vi "Find Region Indices.vi"(11 "Spreadsheet Array":string[][](array[string])) -> (0 "UES Index":i32[](array[numeric]), 1 "Hypo Index":i32[](array[numeric]), 2 "Tongue Index":i32[](array[numeric]), 3 "Velo Index":i32[](array[numeric]))   [LabVIEW 2020]
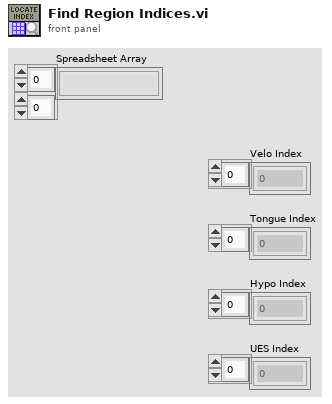
[diagram p1: front panel]
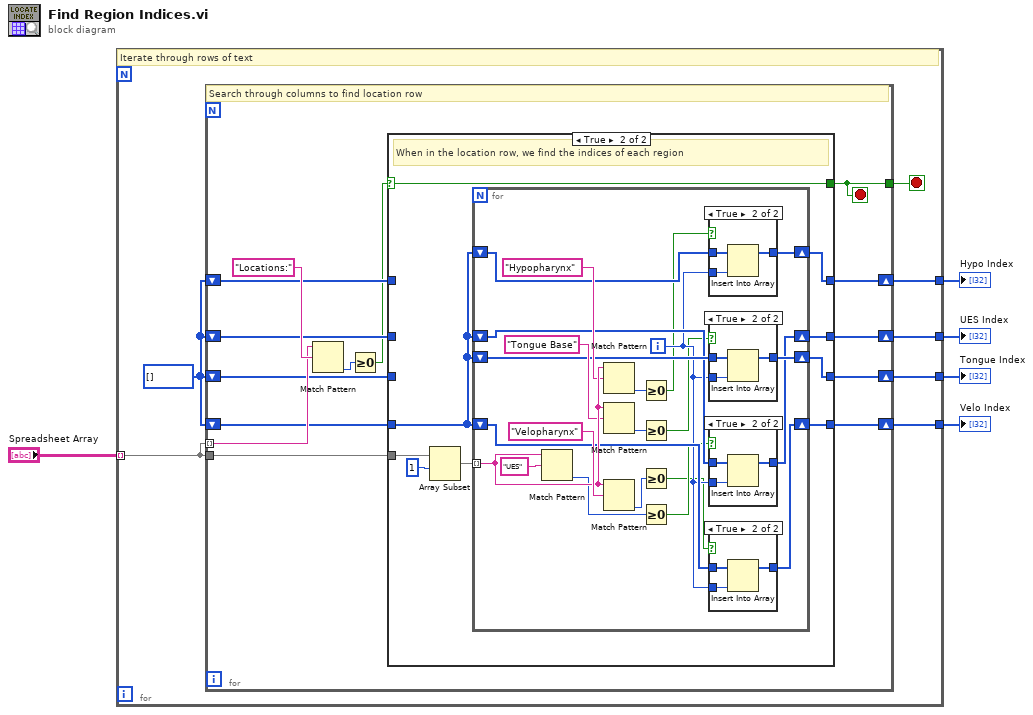
[diagram p0: block diagram]
diagram:
  n1 = for {
    tunnel: [w12] -> w5
    tunnel: [w11] -> w4
    tunnel: [w10] -> w3
    tunnel: [w9] -> w2
    tunnel: "Spreadsheet Array" -> [w7] mode=indexing
    stop <- w6 stop-if-true
    w8 = i32[] [] ("array")
    # "Iterate through rows of text"
    n2 = for {
      tunnel: w7 -> [w24] mode=indexing
      tunnel: w7 -> [w14]
      shift-right: [w19] -> w9
      shift-left: w8 -> [w23]
      shift-right: [w20] -> w12
      shift-left: w8 -> [w16]
      shift-right: [w21] -> w11
      shift-left: w8 -> [w17]
      shift-right: [w22] -> w10
      shift-left: w8 -> [w18]
      tunnel: [w13] -> w6
      stop <- w13 stop-if-true
      # "Search through columns to find location row"
      n3 = Match Pattern(string=w24, regular expression="Locations:" ("element")) -> (offset past match=w25:i32)  [unwired: 1 in, 3 out]
      n4 = Greater Or Equal To 0?(x=w25) -> (x >= 0?=w15:bool)
      n5 = case shown="True" w15 {
        selector: w15 -> [w27 w32]
        tunnel: w14 -> [_ w34]
        tunnel: w23 -> [w31 w40]
        tunnel: [w31 w39] -> w19
        tunnel: [w30 w38] -> w22
        tunnel: [w29 w37] -> w21
        tunnel: [w28 w36] -> w20
        tunnel: w18 -> [w30 _]
        tunnel: w17 -> [w29 _]
        tunnel: w16 -> [w28 _]
        tunnel: [w27 w32] -> w13
        frame False {
        }
        frame True {
          # "When in the location row, we find the indices of each region"
          n6 = Array Subset(array=w34, index=1) -> (w33:string[])  [unwired: 1 in]
          n7 = for {
            tunnel: w33 -> [w61] mode=indexing
            shift-right: [w55] -> w39
            shift-left: w40 -> [w56]
            shift-right: [w47] -> w38
            shift-left: w40 -> [w51]
            shift-right: [w46] -> w37
            shift-left: w40 -> [w50]
            shift-right: [w45] -> w36
            shift-left: w40 -> [w49]
            i -> [w48]
            n8 = Match Pattern(string=w61, regular expression="UES") -> (offset past match=w53:i32)  [unwired: 1 in, 3 out]
            n9 = Match Pattern(string=w61, regular expression="Hypopharynx") -> (offset past match=w52:i32)  [unwired: 1 in, 3 out]
            n10 = Match Pattern(string=w61, regular expression="Tongue Base") -> (offset past match=w54:i32)  [unwired: 1 in, 3 out]
            n11 = Match Pattern(string=w61, regular expression="Velopharynx") -> (offset past match=w57:i32)  [unwired: 1 in, 3 out]
            n12 = Greater Or Equal To 0?(x=w52) -> (x >= 0?=w43:bool)
            n13 = Greater Or Equal To 0?(x=w54) -> (x >= 0?=w44:bool)
            n14 = Greater Or Equal To 0?(x=w57) -> (x >= 0?=w41:bool)
            n15 = Greater Or Equal To 0?(x=w53) -> (x >= 0?=w42:bool)
            n16 = case shown="True" w43 {
              tunnel: w48 -> [_ w70]
              tunnel: w50 -> [w67 w69]
              tunnel: [w67 w68] -> w46
              frame False {
              }
              frame True {
                n17 = Insert Into Array(array=w69, new element=w70) -> (w68:i32[])  [unwired: 1 in]
              }
            }
            n18 = case shown="True" w44 {
              tunnel: w48 -> [_ w74]
              tunnel: w51 -> [w71 w73]
              tunnel: [w71 w72] -> w47
              frame False {
              }
              frame True {
                n19 = Insert Into Array(array=w73, new element=w74) -> (w72:i32[])  [unwired: 1 in]
              }
            }
            n20 = case shown="True" w42 {
              tunnel: w48 -> [_ w66]
              tunnel: w49 -> [w63 w65]
              tunnel: [w63 w64] -> w45
              frame False {
              }
              frame True {
                n21 = Insert Into Array(array=w65, new element=w66) -> (w64:i32[])  [unwired: 1 in]
              }
            }
            n22 = case shown="True" w41 {
              tunnel: w48 -> [_ w78]
              tunnel: w56 -> [w75 w77]
              tunnel: [w75 w76] -> w55
              frame False {
              }
              frame True {
                n23 = Insert Into Array(array=w77, new element=w78) -> (w76:i32[])  [unwired: 1 in]
              }
            }
          }
        }
      }
    }
  }
  "UES Index" <- w5
  "Hypo Index" <- w4
  "Tongue Index" <- w3
  "Velo Index" <- w2
